vi "get Pump Version.vi"(7 "miscVersion":i32, 8 "error in (no error)":errorcluster, 9 "minorVersion":i32, 10 "majorVersion":i32, 11 "pumpIndex":u32) -> (0 "error out":errorcluster, 1 "minorVersion out":i32, 2 "majorVersion out":i32, 3 "function return":i32, 5 "miscVersion out":i32)   [LabVIEW 2018, in "AsiaPumpInterface.lvlib"]
doc: "extern ASIAPUMP_INTERFACE_API BOOL getPumpVersion( unsigned int pumpIndex ,\n int * majorVersion ,\n int * minorVersion ,\n int * miscVersion );"
uses:
  <userlib>/AsiaPumpInterface/AsiaPumpInterface.lvlib
  <userlib>/AsiaPumpInterface/AsiaPumpInterface.dll
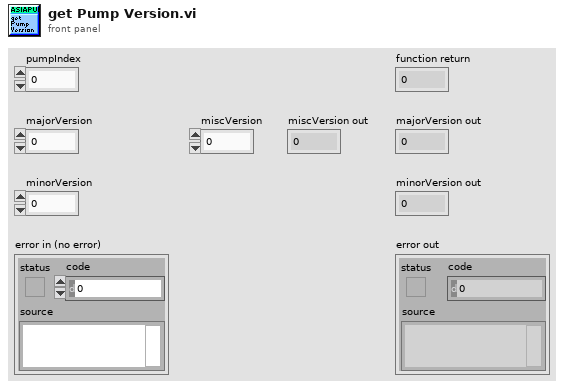
[diagram p1: front panel]
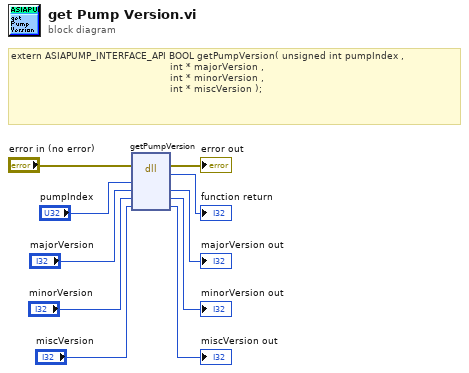
[diagram p0: block diagram]
diagram:
  # "extern ASIAPUMP_INTERFACE_API BOOL getPumpVersion( unsigned int pumpIndex ,\n                                                     int * majorVersion ,\n                                                     int * minorVersion ,\n                                                     int * miscVersion );"
  n1 = dll-call lib="C:/Program Files (x86)/National Instruments/LabVIEW 2018/user.lib/AsiaPumpInterface/AsiaPumpInterface.*" fn="getPumpVersion"(error in="error in (no error)", "pumpIndex"="pumpIndex", "majorVersion"="majorVersion", "minorVersion"="minorVersion", "miscVersion"="miscVersion") -> (error out=→"error out":errorcluster, →"function return":i32, "majorVersion"=→"majorVersion out":i32, "minorVersion"=→"minorVersion out":i32, "miscVersion"=→"miscVersion out":i32)  [unwired: 3 in, 1 out]
